vi "Load.vi"(8 "error in (no error)":errorcluster) -> (0 "error out":errorcluster)   [LabVIEW 2020, in "WebServiceImporter.lvlib" / "Main Panel.lvlib" / "Select Methods.lvlib"]
uses:
  <vilib>/Platform/WebService/Main Panel/Pages/Select Methods/Select Methods.lvlib
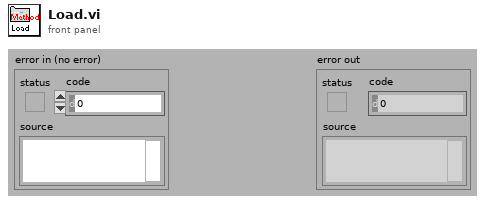
[diagram p1: front panel]
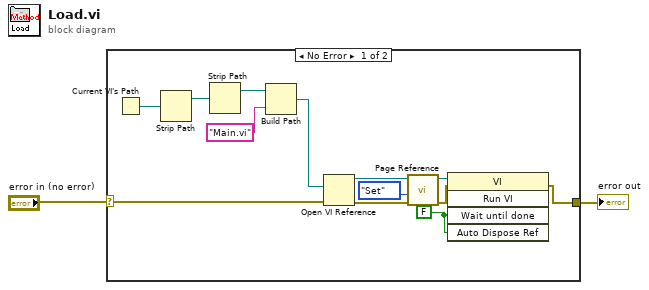
[diagram p0: block diagram]
diagram:
  n1 = case shown="No Error" "error in (no error)" {
    selector: "error in (no error)" -> [w8 w16]
    tunnel: [w4 w16] -> w1
    frame No Error {
      w3 = FALSE ("Wait Until Done")
      n2 = Current VI's Path() -> (path=w15:path)
      n3 = Strip Path(path=w15) -> (stripped path=w14:path)  [unwired: 1 out]
      n4 = Strip Path(path=w14) -> (stripped path=w13:path)  [unwired: 1 out]
      n5 = Build Path(base path=w13, name or relative path="Main.vi") -> (appended path=w11:path)
      n6 = Open VI Reference(vi path=w11, error in (no error)=w8) -> (vi reference=w9:refnum<vi>, error out=w7:errorcluster)  [unwired: 4 in]
      n7 = call <vilib>:"Page Reference.vi"("error in (no error)"=w7, "Operation"=enum16{"Get", "Set"}."Set", "VI Refnum"=w9) -> ("error out"=w6:errorcluster, "VI Refnum (out)"=w5:refnum<vi>)  [unwired: 7 in]
      n8 = invoke class="VI" method="Run VI"(reference=w5, error in=w6, "Wait until done"=w3, "Auto Dispose Ref"=w3) -> (error out=w4:errorcluster)  [unwired: 1 in, 4 out]
    }
    frame Error {
    }
  }
  "error out" <- w1
